vi "Create Column Definition.vi"(6 "Column Definition":T1, 8 "error in (no error)":errorcluster, 10 "GridColumn in":refnum<class "GridColumn.lvclass">) -> (0 "error out":errorcluster, 2 "GridColumn out":refnum<class "GridColumn.lvclass">)   [LabVIEW 2014, in "GridColumn.lvclass"]
uses:
  GridColumn.lvclass
  GridColumn.lvclass/GridColumn.ctl
  Write Name.vi
  Write datatype.vi
  Write Params.vi
  Write AutoSizeMode.vi
  Write FillWeight.vi
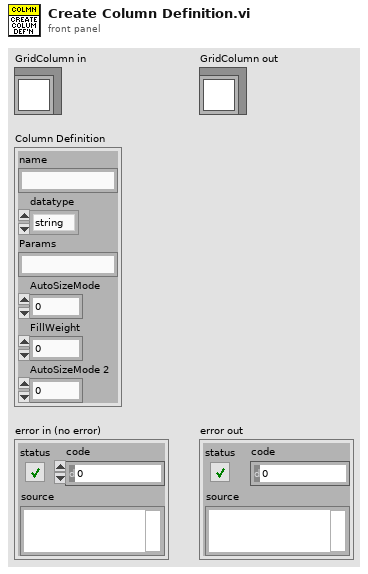
[diagram p1: front panel]
types:
  T1 = cluster{"name":string, "datatype":enum16{"string", "image", "link", "check", "combo", "button"}, "Params":string, "AutoSizeMode":i32, "FillWeight":sgl, "AutoSizeMode 2":i32}
  T2 = enum16{"string", "image", "link", "check", "combo", "button"}
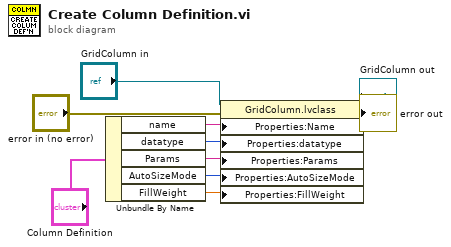
[diagram p0: block diagram]
diagram:
  n1 = Unbundle By Name("Column Definition") -> ("name"=w6:string, "datatype"=w7:T2, "Params"=w8:string, "AutoSizeMode"=w9:i32, "FillWeight"=w10:sgl)
  n2 = property class="GridColumn.lvclass"(reference="GridColumn in", error in="error in (no error)", "Properties:Name"=w6, "Properties:datatype"=w7, "Properties:Params"=w8, "Properties:AutoSizeMode"=w9, "Properties:FillWeight"=w10) -> (reference out=→"GridColumn out":refnum<class "GridColumn.lvclass">, error out=→"error out":errorcluster)
